vi "IsEmptyObject.vi"(3 "error in (no error)":errorcluster, 5 "reference in":refnum<class "G#Object.lvclass">) -> (0 "error out":errorcluster, 1 "is empty?":bool, 2 "reference out":refnum<class "G#Object.lvclass">)   [LabVIEW 2017, in "G#Object.lvclass"]
doc: "Checks if the reference is of G#Object root type and thereby an empty object."
uses:
  G#Object.lvclass
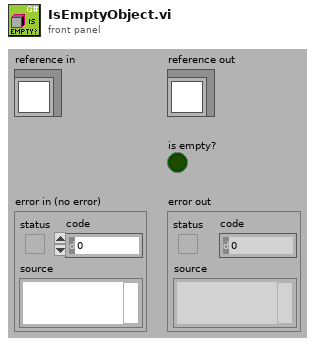
[diagram p1: front panel]
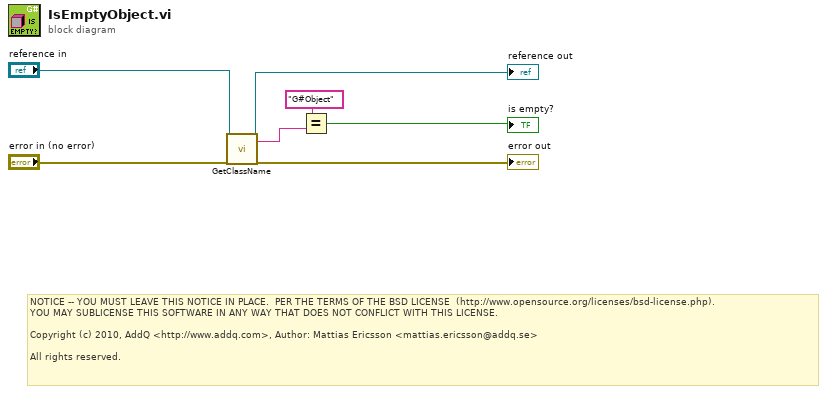
[diagram p0: block diagram]
diagram:
  # "NOTICE -- YOU MUST LEAVE THIS NOTICE IN PLACE.  PER THE TERMS OF THE BSD LICENSE  (http://www.opensource.org/licenses/bsd-license.php).\nYOU MAY SUBLICENSE THIS SOFTWARE IN ANY WAY THAT DOES NOT CONFLICT WITH THIS LICENSE.\n\nCopyright (c) 2010, AddQ <http://www.addq.com>, Author: Mattias Ericsson <mattias.ericsson@addq.se>\n\nAll rights reserved."
  n1 = call-dynamic "GetClassName.vi"("reference in"="reference in", "error in (no error)"="error in (no error)") -> ("reference out"=→"reference out":refnum<class "G#Object.lvclass">, "class name"=w6:string, "error out"=→"error out":errorcluster)  [unwired: 13 in, 2 out]
  n2 = Equal?(x="G#Object", y=w6) -> (x = y?=→"is empty?":bool)
